vi "_Serial Port-Initialize.vi"(4 "baud rate":u32=9600, 5 "Serial Port":refnum<visa-resource-name>="COM3") -> (1 "Serial Port 2":refnum<visa-resource-name>="COM3", 2 "Normal":bool)   [LabVIEW 2015]
uses:
  <vilib>/Instr/_visa.llb/VISA Configure Serial Port (Instr).vi
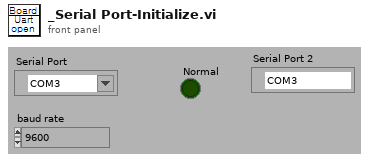
[diagram p1: front panel]
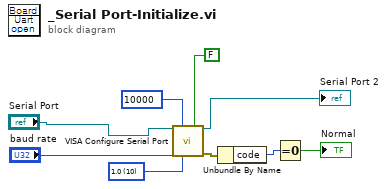
[diagram p0: block diagram]
diagram:
  w6 = u16 10 items=["1.0"=10, "1.5"=15, "2.0"=20] ("stop bits (10: 1 bit)")
  n1 = call-poly "VISA Configure Serial Port"("VISA resource name"="Serial Port", "timeout (10sec)"=u32 10000, "Enable Termination\nChar (T)"=FALSE ("Enable Termination\nChar (T)"), "baud rate (9600)"="baud rate", "stop bits (10: 1 bit)"=w6) -> ("VISA resource name out"=→"Serial Port 2":refnum<visa-resource-name>, "error out"=w8:errorcluster)  [unwired: 4 in, 5 out]
  n2 = Unbundle By Name(w8) -> ("code"=w7:i32)
  n3 = Equal To 0?(x=w7) -> (x = 0?=→"Normal":bool)
